vi "StartingLocations.vi"(11 "Index":i32) -> (3 "Location":cluster{dbl, dbl})   [LabVIEW 2020]
uses:
  Robot Project/Configuration/Constants.vi
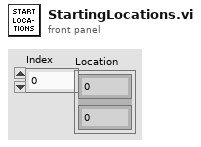
[diagram p1: front panel]
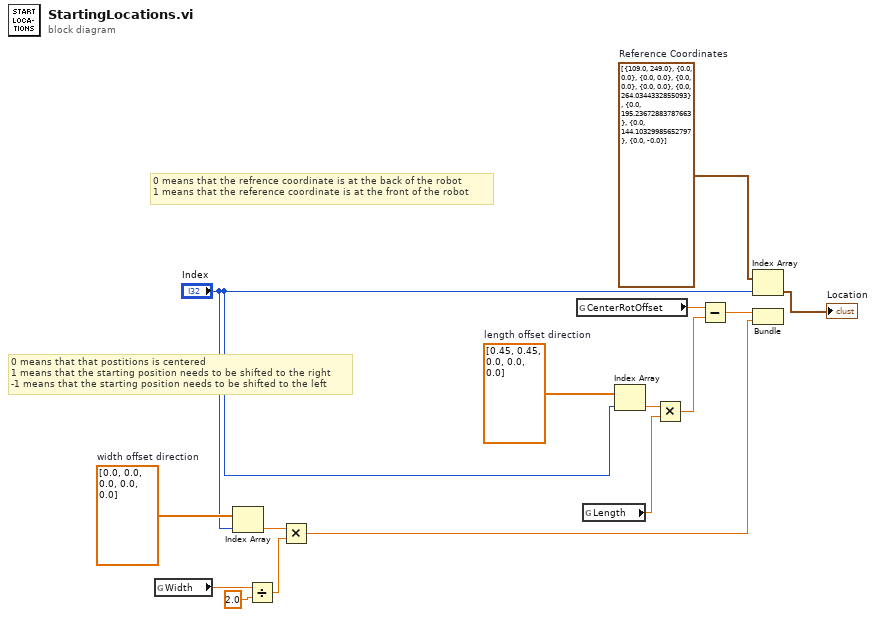
[diagram p0: block diagram]
diagram:
  w6 = dbl[] [0.45, 0.45, 0.0, 0.0, 0.0]  # length offset direction
  w12 = dbl[] [0.0, 0.0, 0.0, 0.0, 0.0]  # width offset direction
  w13 = cluster{dbl, dbl}[] [{109.0, 249.0}, {0.0, 0.0}, {0.0, 0.0}, {0.0, 0.0}, {0.0, 0.0}, {0.0, 264.0344332855093}, {0.0, 195.23672883787663}, {0.0, 144.10329985652797}, {0.0, -0.0}]  # Reference Coordinates
  # "0 means that that postitions is centered\n1 means that the starting position needs to be shifted to the right\n-1 means that the starting position needs to be shifted to the left"
  # "0 means that the refrence coordinate is at the back of the robot\n1 means that the reference coordinate is at the front of the robot"
  n1 = global read "Constants.vi" "Width"() -> (w10:dbl)
  n2 = Index Array(array=w12, index="Index") -> (element=w14:dbl)
  n3 = Divide(x=w10, y=2.0) -> (x/y=w11:dbl)
  n4 = Multiply(x=w14, y=w11) -> (x*y=w15:dbl)
  n5 = global read "Constants.vi" "CenterRotOffset"() -> (w7:dbl)
  n6 = global read "Constants.vi" "Length"() -> (w8:dbl)
  n7 = Index Array(array=w6, index="Index") -> (element=w5:dbl)
  n8 = Multiply(x=w5, y=w8) -> (x*y=w3:dbl)
  n9 = Subtract(x=w7, y=w3) -> (x-y=w2:dbl)
  n10 = Index Array(array=w13, index="Index") -> (element=→"Location":cluster{dbl, dbl})
  n11 = Bundle(w2, w15) -> ()  [unwired: 1 in, 1 out]
